vi "Load Filter Files.vi"(11 "path":path) -> (3 "Array of Filters":T1(array[cluster]))   [LabVIEW 2011]
uses:
  <vilib>/Utility/file.llb/Read From Spreadsheet File (DBL).vi
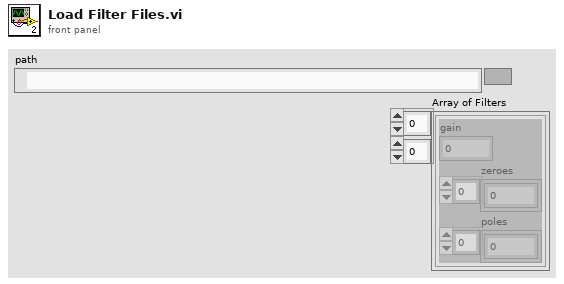
[diagram p1: front panel]
types:
  T1 = cluster{"gain":dbl, "zeroes":cdb[], "poles":cdb[]}[][]
  T2 = cluster{"gain":dbl, "zeroes":cdb[], "poles":cdb[]}
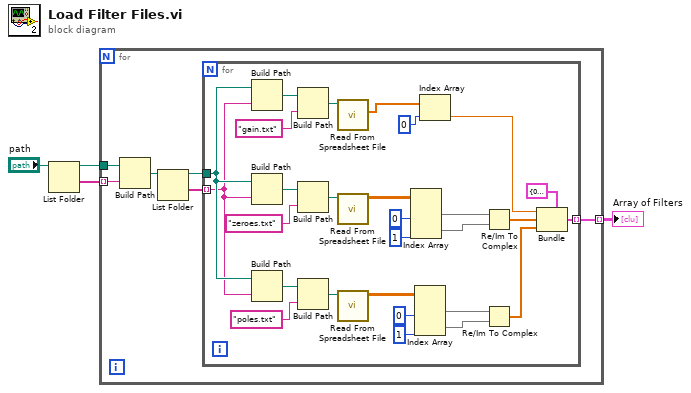
[diagram p0: block diagram]
diagram:
  n1 = List Folder(path="path") -> (path out=w3:path, folder names=w4:string[])  [unwired: 3 in, 2 out]
  n2 = for {
    tunnel: w4 -> [w8] mode=indexing
    tunnel: w3 -> [w9]
    tunnel: [w6] -> w1 mode=indexing
    n3 = Build Path(base path=w9, name or relative path=w8) -> (appended path=w7:path)
    n4 = List Folder(path=w7) -> (path out=w5:path, folder names=w10:string[])  [unwired: 3 in, 2 out]
    n5 = for {
      tunnel: w10 -> [w17] mode=indexing
      tunnel: w5 -> [w18]
      tunnel: [w30] -> w6 mode=indexing
      n6 = Build Path(base path=w18, name or relative path=w17) -> (appended path=w21:path)
      n7 = Build Path(base path=w18, name or relative path=w17) -> (appended path=w35:path)
      n8 = Build Path(base path=w18, name or relative path=w17) -> (appended path=w26:path)
      n9 = Build Path(base path=w21, name or relative path="gain.txt") -> (appended path=w19:path)
      n10 = Build Path(base path=w35, name or relative path="zeroes.txt") -> (appended path=w33:path)
      n11 = Build Path(base path=w26, name or relative path="poles.txt") -> (appended path=w24:path)
      n12 = call-poly <vilib>:"Read From Spreadsheet File.vi"("file path (dialog if empty)"=w19) -> ("first row"=w16:dbl[])  [unwired: 6 in, 4 out]
      n13 = call-poly <vilib>:"Read From Spreadsheet File.vi"("file path (dialog if empty)"=w33) -> ("all rows"=w38:dbl[][])  [unwired: 6 in, 4 out]
      n14 = call-poly <vilib>:"Read From Spreadsheet File.vi"("file path (dialog if empty)"=w24) -> ("all rows"=w29:dbl[][])  [unwired: 6 in, 4 out]
      n15 = Index Array(array=w38, index (col) #1=0 ("disabled index (col)"), index (col) #2=1 ("index (col)")) -> (element #1=w32:dbl[], element #2=w31:dbl[])  [unwired: 2 in]
      n16 = Index Array(array=w29, index (col) #1=0 ("disabled index (col)"), index (col) #2=1 ("index (col)")) -> (element #1=w23:dbl[], element #2=w22:dbl[])  [unwired: 2 in]
      n17 = Index Array(array=w16, index=0 ("disabled index (col)")) -> (element=w11:dbl)
      n18 = Re/Im To Complex(1:w31, 2:w32) -> (0:w12:cdb[])
      n19 = Re/Im To Complex(1:w22, 2:w23) -> (0:w13:cdb[])
      n20 = Bundle(cluster=T2 {"gain"=0.0, "zeroes"=[], "poles"=[]}, "gain"=w11, "zeroes"=w12, "poles"=w13) -> (w30:T2)
    }
  }
  "Array of Filters" <- w1
